vi "getLibraryDirectory.vi"() -> (0 "Library Directory":path)   [LabVIEW 2017, in "Document API.lvlib" / "Document API.lvclass"]
uses:
  Document API.lvclass
  <vilib>/Simplicity AI/SAI_PDF_API/Classes/Context/Context.lvclass
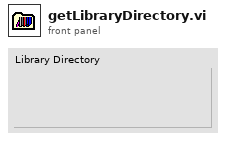
[diagram p1: front panel]
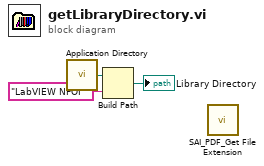
[diagram p0: block diagram]
diagram:
  n1 = call <vilib>:"Application Directory.vi"() -> ("Application Directory"=w3:path)
  n2 = Build Path(base path=w3, name or relative path="LabVIEW NPOI") -> (appended path=→"Library Directory":path)
  n3 = call <vilib>:"SAI_PDF_Get File Extension.vi"() -> ()  [unwired: 11 in, 1 out]
